vi "Read COM.vi"(8 "error in (no error)":errorcluster, 11 "Tektronic in":refnum<class "Tektronic.lvclass">) -> (0 "error out":errorcluster, 2 "COM":refnum<visa-resource-name>, 3 "Tektronic out":refnum<class "Tektronic.lvclass">)   [LabVIEW 2020, in "Controlador.lvlib" / "Tektronic.lvclass"]
uses:
  Tektronic/Tektronic.lvclass
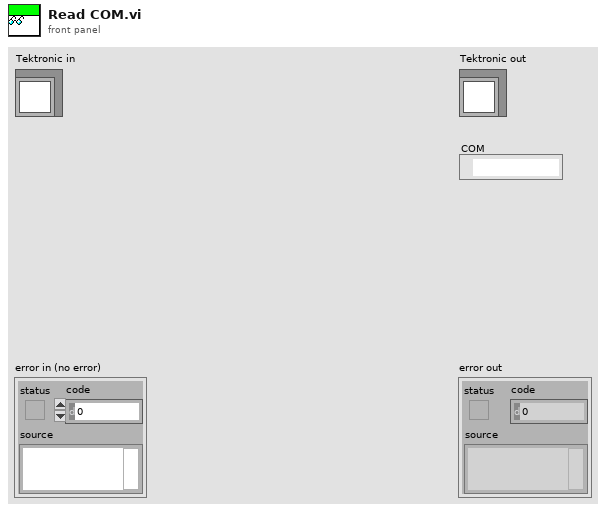
[diagram p1: front panel]
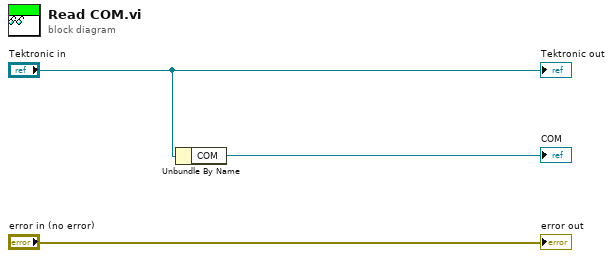
[diagram p0: block diagram]
diagram:
  n1 = Unbundle By Name("Tektronic in") -> ("COM"=→"COM":refnum<visa-resource-name>)
  "error out" <- "error in (no error)"
  "Tektronic out" <- "Tektronic in"
